vi "Main_SubVI_Response to Pulse.vi"(8 "Error In":errorcluster, 11 "Response":string) -> (0 "Error Out":errorcluster, 3 "Pulse":i32)   [LabVIEW 2015]
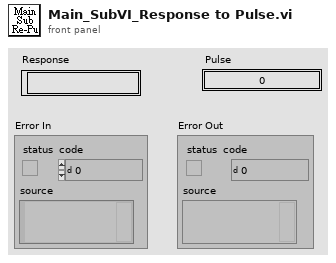
[diagram p1: front panel]
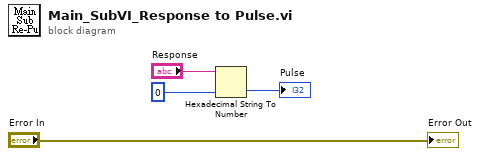
[diagram p0: block diagram]
diagram:
  n1 = Hexadecimal String To Number(string="Response", default (0uL)=0 ("default (0 U32)")) -> (number=→"Pulse":i32)  [unwired: 1 in, 1 out]
  "Error Out" <- "Error In"
